vi "Locate Bracket Holes.vi"() -> ()   [LabVIEW 2013]
panel:
  out "Particle Measurements (Pixels) (Particle Analysis 1)":dbl[][](array[numeric]) format="%.2f"
  out "Number of Particles (Particle Analysis 1)":i32
  out "Image Out":T1(plugin-control)
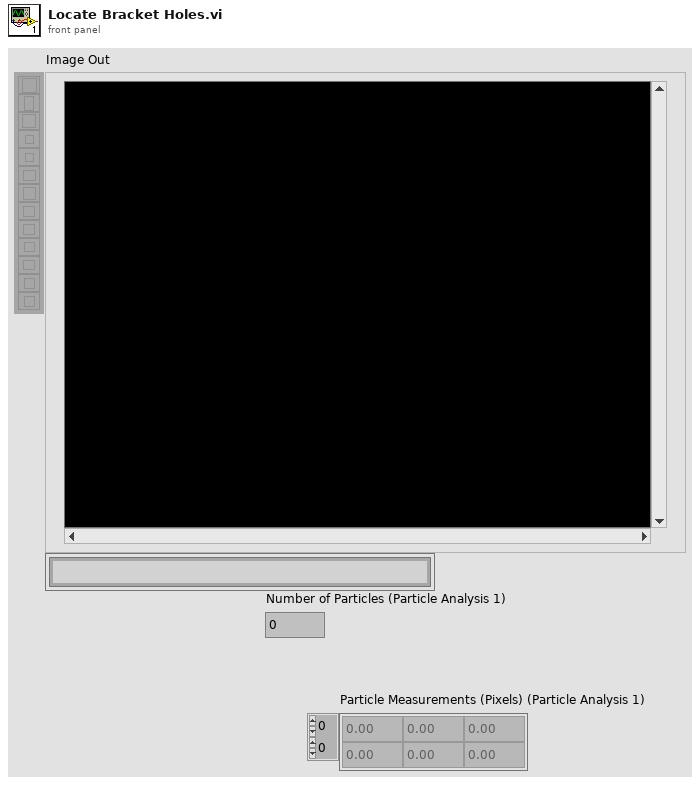
[diagram p1: front panel]
types:
  T1 = typedef "IMAQ Image.ctl" = refnum<image>
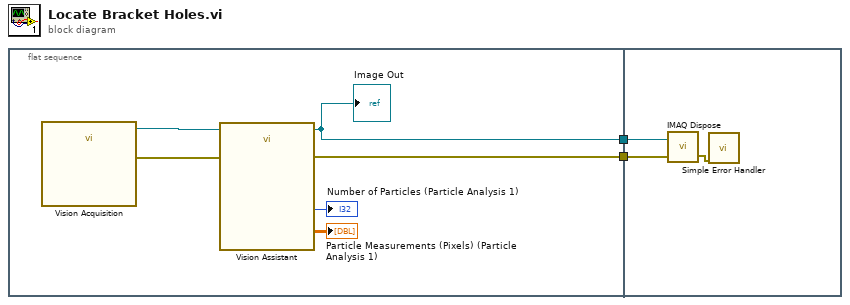
[diagram p0: block diagram]
diagram:
  n1 = flat-sequence {
    tunnel: [w4] -> w2
    tunnel: [w3] -> w1
    tunnel: w2 -> [w11]
    tunnel: w1 -> [w10]
    frame #0 {
      n2 = call "Vision Acquisition"() -> ("Image Out"=w6:T1, "error out"=w5:errorcluster)  [unwired: 26 in]
      n3 = call "Vision Assistant"("Image In"=w6, "error in"=w5) -> ("Image Out"=w3:T1, "Number of Particles (Particle Analysis 1)"=→"Number of Particles (Particle Analysis 1)":i32, "Particle Measurements (Pixels) (Particle Analysis 1)"=→"Particle Measurements (Pixels) (Particle Analysis 1)":dbl[][], "error out"=w4:errorcluster)  [unwired: 22 in]
      "Image Out" <- w3
    }
    frame #1 {
      n4 = call "IMAQ Dispose"("Image"=w10, "error in (no error)"=w11) -> ("error out"=w9:errorcluster)  [unwired: 4 in]
      n5 = call <vilib>:"Simple Error Handler.vi"("error in (no error)"=w9) -> ()  [unwired: 4 in, 5 out]
    }
  }
